vi "add scan harm(SubVI).vi"(10 "字符串":string) -> (1 "ok or cancel":bool=TRUE, 2 "连接的字符串":string)   [LabVIEW 2019, in "Add Seq.lvlib"]
uses:
  Add Seq.lvlib
panel:
  in  "Number of Step":i32=2
  in  "Increments":i32=10
  in  "Final harm":i32
  in  "Initial harm":i32
  in  "cancel":bool
  in  "ok":bool
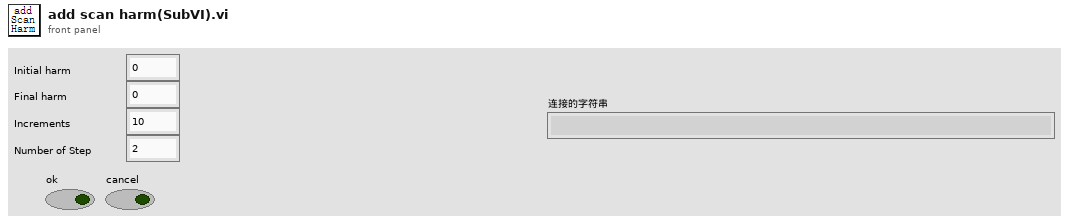
[diagram p1: front panel]
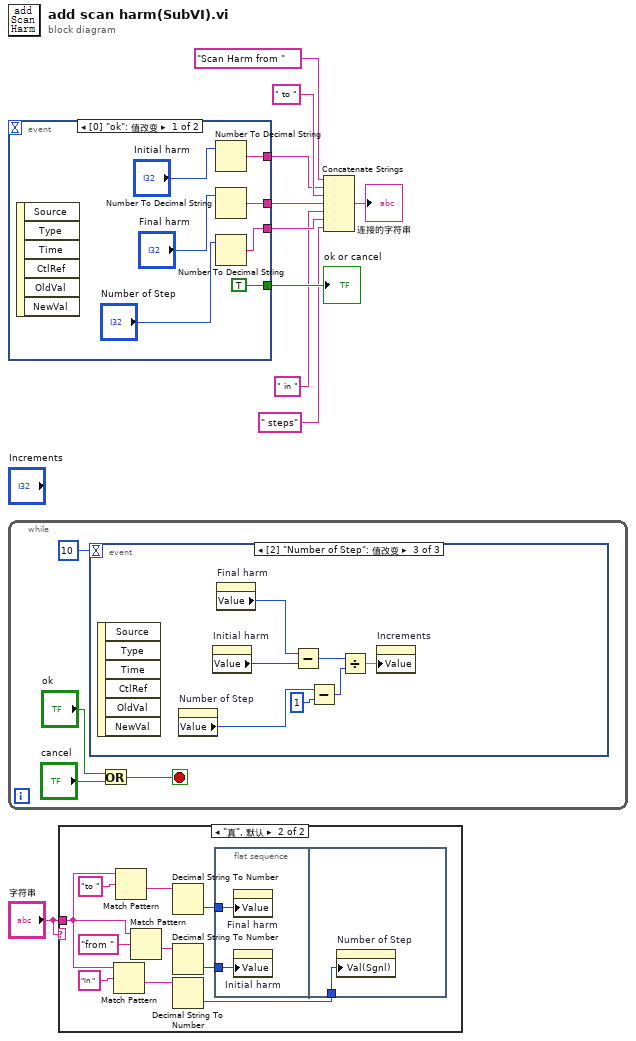
[diagram p0: block diagram]
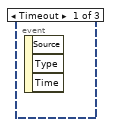
[diagram p3: hidden frame]
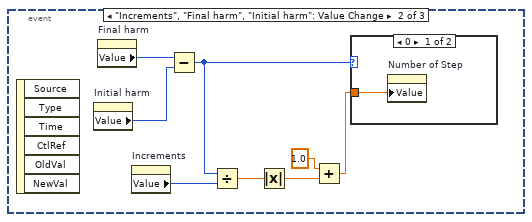
[diagram p4: hidden frame]
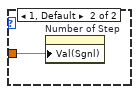
[diagram p5: hidden frame]
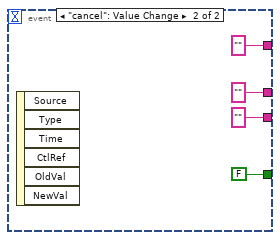
[diagram p6: hidden frame]
diagram:
  n1 = event shown="[0] \"ok\": 值改变" {
    selector: _ -> [_ _]
    dyn-events: _ -> [_ _]
    timeout: _ -> [_ _]
    tunnel: [TRUE FALSE] -> w8
    tunnel: [w15 ""] -> w6
    tunnel: [w11 ""] -> w4
    tunnel: [w13 ""] -> w3
    event "ok": Value Change {
      n2 = event-data() -> ()  [unwired: 1 in, 6 out]
      n3 = Number To Decimal String(number="Initial harm") -> (decimal integer string=w15:string)  [unwired: 1 in]
      n4 = Number To Decimal String(number="Final harm") -> (decimal integer string=w13:string)  [unwired: 1 in]
      n5 = Number To Decimal String(number="Number of Step") -> (decimal integer string=w11:string)  [unwired: 1 in]
    }
    event "cancel": Value Change {
      n6 = event-data() -> ()  [unwired: 1 in, 6 out]
    }
  }
  "ok or cancel" <- w8
  n7 = while {
    stop <- w24 stop-if-true
    n8 = event shown="[2] \"Number of Step\": 值改变" {
      selector: _ -> [_ _ _]
      dyn-events: _ -> [_ _ _]
      timeout: 10 -> [_ _ _]
      event Timeout {
        n9 = event-data() -> ()  [unwired: 1 in, 3 out]
      }
      event "Increments", "Final harm", "Initial harm": Value Change {
        n10 = event-data() -> ()  [unwired: 1 in, 6 out]
        n11 = property on="Initial harm" class="DigNum (严格)"() -> ("Value"=w29:i32)  [unwired: 2 in, 2 out]
        n12 = property on="Final harm" class="DigNum (严格)"() -> ("Value"=w30:i32)  [unwired: 2 in, 2 out]
        n13 = property on="Increments" class="DigNum (严格)"() -> ("Value"=w28:i32)  [unwired: 2 in, 2 out]
        n14 = Subtract(x=w30, y=w29) -> (x-y=w26:i32)
        n15 = Divide(x=w26, y=w28) -> (x/y=w32:dbl)
        n16 = Absolute Value(x=w32) -> (abs(x)=w31:dbl)
        n17 = Add(x=1.0, y=w31) -> (x+y=w27:dbl)
        n18 = case shown="0" w26 {
          tunnel: w27 -> [w34 w35]
          frame 0 {
            n19 = property on="Number of Step" class="DigNum (严格)"("Value"=w34) -> ()  [unwired: 2 in, 2 out]
          }
          frame 1, Default {
            n20 = property on="Number of Step" class="DigNum (严格)"("Val(Sgnl)"=w35) -> ()  [unwired: 2 in, 2 out]
          }
        }
      }
      event "Number of Step": Value Change {
        n21 = event-data() -> ()  [unwired: 1 in, 6 out]
        n22 = property on="Number of Step" class="DigNum (严格)"() -> ("Value"=w37:i32)  [unwired: 2 in, 2 out]
        n23 = property on="Initial harm" class="DigNum (严格)"() -> ("Value"=w38:i32)  [unwired: 2 in, 2 out]
        n24 = property on="Final harm" class="DigNum (严格)"() -> ("Value"=w39:i32)  [unwired: 2 in, 2 out]
        n25 = Subtract(x=w39, y=w38) -> (x-y=w42:i32)
        n26 = Subtract(x=w37, y=1) -> (x-y=w40:i32)
        n27 = Divide(x=w42, y=w40) -> (x/y=w36:dbl)
        n28 = property on="Increments" class="DigNum (严格)"("Value"=w36) -> ()  [unwired: 2 in, 2 out]
      }
    }
    n29 = Or(x="ok", y="cancel") -> (x .or. y?=w24:bool)
  }
  n30 = case shown="\"真\", 默认" "字符串" {
    tunnel: "字符串" -> [_ w45]
    frame "" {
    }
    frame "真", Default {
      n31 = Match Pattern(string=w45, regular expression="in " ("正则表达式")) -> (after substring=w50:string)  [unwired: 1 in, 3 out]
      n32 = Match Pattern(string=w45, regular expression="to " ("正则表达式")) -> (after substring=w43:string)  [unwired: 1 in, 3 out]
      n33 = Match Pattern(string=w45, regular expression="from " ("正则表达式")) -> (after substring=w46:string)  [unwired: 1 in, 3 out]
      n34 = Decimal String To Number(string=w43) -> (number=w48:i32)  [unwired: 2 in, 1 out]
      n35 = Decimal String To Number(string=w46) -> (number=w49:i32)  [unwired: 2 in, 1 out]
      n36 = Decimal String To Number(string=w50) -> (number=w47:i32)  [unwired: 2 in, 1 out]
      n37 = flat-sequence {
        tunnel: w49 -> [w54]
        tunnel: w48 -> [w53]
        tunnel: w47 -> [w55]
        frame #0 {
          n38 = property on="Final harm" class="DigNum (严格)"("Value"=w53) -> ()  [unwired: 2 in, 2 out]
          n39 = property on="Initial harm" class="DigNum (严格)"("Value"=w54) -> ()  [unwired: 2 in, 2 out]
        }
        frame #1 {
          n40 = property on="Number of Step" class="DigNum (严格)"("Val(Sgnl)"=w55) -> ()  [unwired: 2 in, 2 out]
        }
      }
    }
  }
  n41 = Concatenate Strings("Scan Harm from " ("字符串"), w6, " to " ("字符串"), w3, " in " ("字符串"), w4, " steps" ("字符串")) -> (→"连接的字符串":string)
